vi "[Map] Filter Entries By Key.vi"(8 "error in (no error)":errorcluster, 10 "Key Filter":string, 11 "Map in":map{string, i32}(c390)) -> (0 "Error Out":errorcluster, 3 "Map out":map{string, i32}(c390))   [LabVIEW 2019]
doc: "Filters a map and returns a new map that only contains entries that match the filter.\n\nThe filter is implemented as a regex whole word match (i.e. the string is placed between two \\b characters)."
uses:
  <vilib>/regexp/Match Regular Expression.xnode
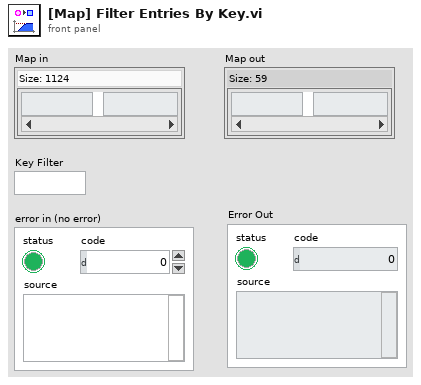
[diagram p1: front panel]
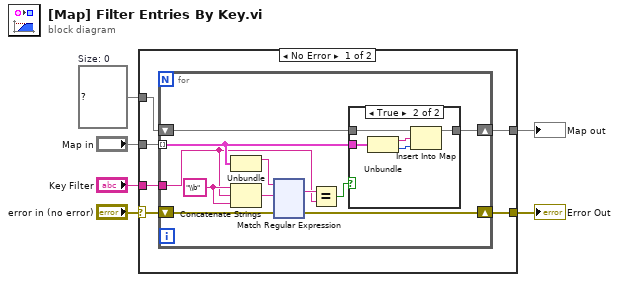
[diagram p0: block diagram]
diagram:
  w6 = map{string, i32} {}  # Size: 0
  n1 = case shown="No Error" "error in (no error)" {
    selector: "error in (no error)" -> [w7 w144]
    tunnel: w6 -> [w12 w145]
    tunnel: "Map in" -> [w11 _]
    tunnel: [w10 w145] -> w4
    tunnel: "Key Filter" -> [w9 _]
    tunnel: [w8 w144] -> w2
    frame No Error {
      n2 = for {
        tunnel: w11 -> [w18] mode=indexing
        shift-right: [w22] -> w8
        shift-left: w7 -> [w21]
        tunnel: w9 -> [w13]
        shift-right: [w17] -> w10
        shift-left: w12 -> [w19]
        w14 = "\\b" ("string")
        n3 = Unbundle(w18) -> (w23:string)  [unwired: 1 out]
        n4 = Concatenate Strings(w14, w13, w14) -> (w15:string)
        n5 = xnode "Match Regular Expression"("input string"=w23, "regular expression"=w15, "error in"=w21) -> ("whole match"=w20:string, "error out"=w22:errorcluster)  [unwired: 3 in, 3 out]
        n6 = Equal?(x=w20, y=w13) -> (x = y?=w16:bool)
        n7 = case shown="True" w16 {
          tunnel: w19 -> [w24 w28]
          tunnel: w18 -> [_ w29]
          tunnel: [w24 w27] -> w17
          frame False {
          }
          frame True {
            n8 = Unbundle(w29) -> (w26:string, w25:i32)
            n9 = Insert Into Map(map in=w28, key=w26, value=w25) -> (map out=w27:map{string, i32})  [unwired: 2 out]
          }
        }
      }
    }
    frame Error {
    }
  }
  "Map out" <- w4
  "Error Out" <- w2
